vi "Read PID Settings.vi"(8 "error in (no error)":errorcluster, 11 "Boot Loader in":refnum<class "Boot Loader.lvclass">) -> (0 "error out":errorcluster, 2 "PID Settings":T1={"Pressure Servo Valve Settings"={"P"=1.0, "I"=0.1, "D"=0.0, "Minimum"=0.0, "Maximum"=10.0}, "Turbo Valve Settings"={"P"=1.0, "I"=0.1, "D"=0.0, "Minimum"=0.0, "Maximum"=10.0}} {"Turbo Valve Settings"."Maximum" format="%.6f"; "Turbo Valve Settings"."Minimum" format="%.6f"; "Turbo Valve Settings"."D" format="%.6f"; "Turbo Valve Settings"."I" format="%.6f"; "Turbo Valve Settings"."P" format="%.6f"; "Pressure Servo Valve Settings"."Maximum" format="%.6f"; "Pressure Servo Valve Settings"."Minimum" format="%.6f"; "Pressure Servo Valve Settings"."D" format="%.6f"; "Pressure Servo Valve Settings"."I" format="%.6f"; "Pressure Servo Valve Settings"."P" format="%.6f"}, 3 "Boot Loader out":refnum<class "Boot Loader.lvclass">)   [LabVIEW 2015, in "Boot Loader.lvclass"]
uses:
  Boot Loader.lvclass
  Typedefs/PID Settings.ctl
  Typedefs/Closed Loop Settings.ctl
  Settings/Settings.lvclass
  Typedefs/FAMT Typedefs.lvlib
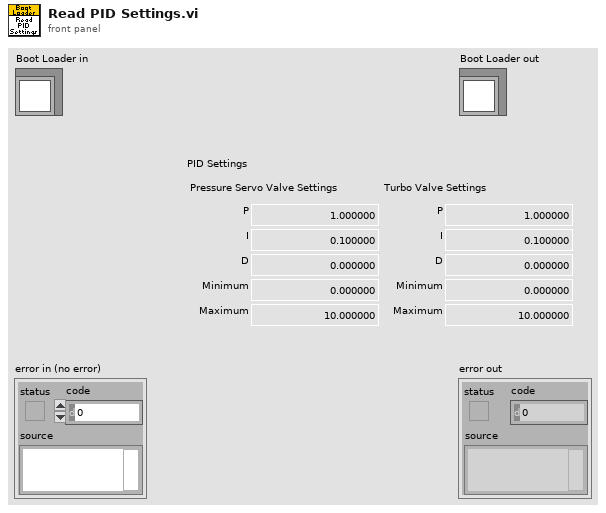
[diagram p1: front panel]
types:
  T1 = typedef "FAMT Typedefs.lvlib/PID Settings.ctl" = cluster{"Pressure Servo Valve Settings":T2, "Turbo Valve Settings":T2}
  T2 = typedef "FAMT Typedefs.lvlib/Closed Loop Settings.ctl" = cluster{"P":dbl, "I":dbl, "D":dbl, "Minimum":dbl, "Maximum":dbl}
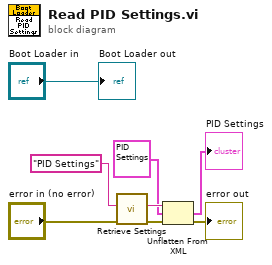
[diagram p0: block diagram]
diagram:
  n1 = call "Retrieve Settings.vi"("error in (no error)"="error in (no error)", "configName"="PID Settings") -> ("error out"=w4:errorcluster, "xmlConfig"=w7:string)  [unwired: 7 in, 1 out]
  n2 = Unflatten From XML(xml string=w7, type=T1 {"Pressure Servo Valve Settings"={"P"=1.0, "I"=0.1, "D"=0.0, "Minimum"=0.0, "Maximum"=10.0}, "Turbo Valve Settings"={"P"=1.0, "I"=0.1, "D"=0.0, "Minimum"=0.0, "Maximum"=10.0}} ("PID Settings"), error in (no error)=w4) -> (value=→"PID Settings":T1, error out=→"error out":errorcluster)
  "Boot Loader out" <- "Boot Loader in"
